vi "Stop.vi"(7 "Write?":bool, 8 "error in (no error)":errorcluster, 10 "StateIn":bool) -> (0 "error out":errorcluster, 2 "StateOut":bool)   [LabVIEW 2018]
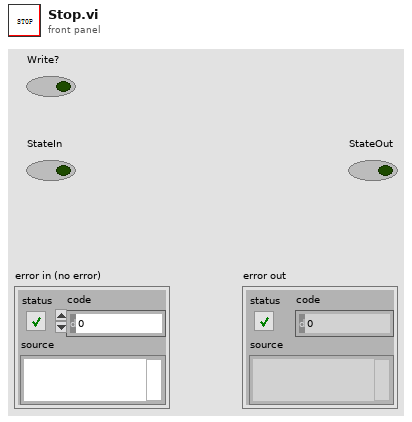
[diagram p1: front panel]
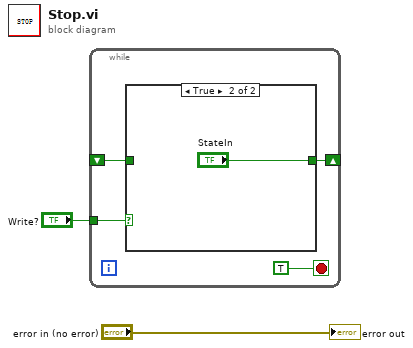
[diagram p0: block diagram]
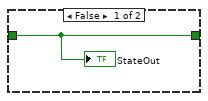
[diagram p2: hidden frame]
diagram:
  n1 = while {
    tunnel: "Write?" -> [w5]
    shift-right: [w4] -> _
    shift-left: _ -> [w3]
    stop <- TRUE stop-if-true
    n2 = case shown="True" w5 {
      tunnel: [w7 "StateIn"] -> w4
      tunnel: w3 -> [w7 _]
      frame False {
        "StateOut" <- w7
      }
      frame True {
      }
    }
  }
  "error out" <- "error in (no error)"
